vi "Pixel Mapping.vi"(8 "error in (no error)":errorcluster, 10 "Pixel Mapping":bool, 11 "Controller in":refnum<class "Controller.lvclass">) -> (0 "error out":errorcluster, 3 "Controller out":refnum<class "Controller.lvclass">)   [LabVIEW 2022 SP3, in "Controller.lvlib" / "Controller.lvclass"]
uses:
  Controller.lvclass
  Controller.lvclass/Controller.ctl
  ImageHandler/ImageHandler Messages/Pixel Map Msg/Pixel Map Msg.lvclass
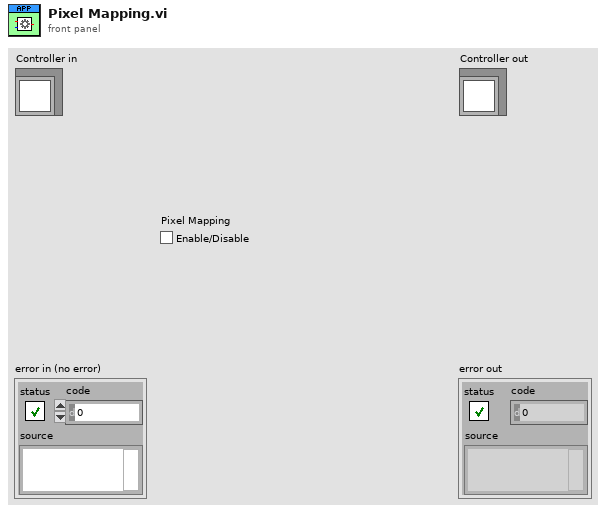
[diagram p1: front panel]
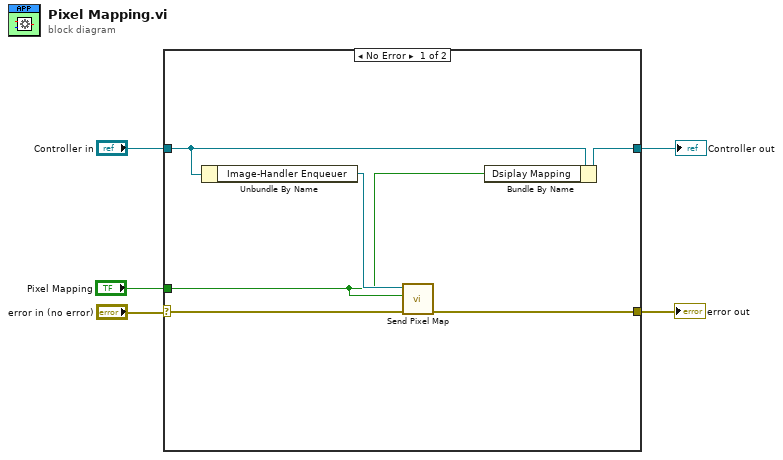
[diagram p0: block diagram]
diagram:
  n1 = case shown="No Error" "error in (no error)" {
    selector: "error in (no error)" -> [w11 w12]
    tunnel: "Controller in" -> [w8 w13]
    tunnel: [w9 w12] -> w3
    tunnel: [w10 w13] -> w2
    tunnel: "Pixel Mapping" -> [w6 _]
    frame No Error {
      n2 = Unbundle By Name(w8) -> ("Image-Handler Enqueuer"=w7:refnum<class "Message Enqueuer.lvclass">)
      n3 = call "Send Pixel Map.vi"("error in (no error)"=w11, "Pixel Map"=w6, "Message Enqueuer"=w7) -> ("error out"=w9:errorcluster)  [unwired: 7 in, 1 out]
      n4 = Bundle By Name(cluster=w8, "Dsiplay Mapping"=w6) -> (w10:refnum<class "Controller.lvclass">)
    }
    frame Error {
    }
  }
  "error out" <- w3
  "Controller out" <- w2
